vi "M2p_AD_Std_Simple.vi"() -> ()   [LabVIEW 2015]
uses:
  spcm_library/spcm_gui_common.llb/element_device.ctl
  spcm_library/spcm_gui_m2p.llb/element_m2p_ad_std.ctl
  spcm_library/spcm_gui_m2p.llb/element_m2p_ai_channel.ctl
  spcm_library/spcm_gui_common.llb/element_mode.ctl
  spcm_library/spcm_gui_m2p.llb/element_m2p_clock.ctl
  spcm_library/spcm_gui_m2p.llb/element_m2p_ai_trigger.ctl
  spcm_library/spcm_gui_m2p.llb/element_m2p_ai_multi_purpose_io.ctl
  spcm_library/spcm_gui_common.llb/element_device_infos.ctl
panel:
  out "Device Infos":T1={"Device Name"="M4i.4451-Exp", "Serial Number"=1122.0, "Mem (MB)"=4096.0}
  out "Display Data":dbl[][](graph)
  in  "M2p AD Settings":T2={"AI Channel 0"={"Enable"=TRUE, "Input Range "=2, "Termination"=0, "Input Type"=0, "Offset"=0}, "AI Channel 1"={"Enable"=TRUE, "Input Range "=2, "Termination"=0, "Input Type"=0, "Offset"=0}, "AI Channel 2"={"Enable"=TRUE, "Input Range "=2, "Termination"=0, "Input Type"=0, "Offset"=0}, "AI Channel 3"={"Enable"=TRUE, "Input Range "=2, "Termination"=0, "Input Type"=0, "Offset"=0}, "AI Channel 4"={"Enable"=TRUE, "Input Range "=2, "Termination"=0, "Input Type"=0, "Offset"=0}, "AI Channel 5"={"Enable"=TRUE, "Input Range "=2, "Termination"=0, "Input Type"=0, "Offset"=0}, "AI Channel 6"={"Enable"=TRUE, "Input Range "=2, "Termination"=0, "Input Type"=0, "Offset"=0}, "AI Channel 7"={"Enable"=TRUE, "Input Range "=2, "Termination"=0, "Input Type"=0, "Offset"=0}, "Mode Setup"={"Mode"=0, "Mem"=16384, "Seg"=1024, "Post"=8192, "Pre"=32, "ABA"=16}, "Clock Settings"={"Clock Mode"=0, "Sampling Rate (kHz)"=10000.0, "Clock Output"=FALSE, "Termination"=FALSE, "Ref. Clock (MHz)"=10.0, "Threshold (mV)"=1500}, "Trigger Settings"={"Trigger Source"=0, "External Trigger"=0, "Level 0 Ext"=1500, "Ext Trig Term"=FALSE, "Channel Trigger"=0, "Level 0 Ch"=0, "Level 1 Ch"=0, "Trigger Delay (Samples)"=0}, "Multi Purpose IO Lines"={"X0 Mode"=0, "X1 Mode"=0, "X2 Mode"=0, "X3 Mode"=0, "X0 ASync Send Pulse"=FALSE, "X1 ASync Send Pulse"=FALSE, "X2 ASync Send Pulse"=FALSE, "X3 ASync Send Pulse"=FALSE, "X1 Trigger Mode"=0, "X2 Trigger Mode"=0, "X3 Trigger Mode"=0, "X1 Pulsewidth"=0, "X2 Pulsewidth"=0, "X3 Pulsewidth"=0, "ASync Read Button"=FALSE, "ASync Read"=0, "AI"=TRUE}} {"Multi Purpose IO Lines"."X3 Mode" items=["Disable", "Asynchronous Out", "Asynchronous In", "Trigger Out", "Trigger In", "Clock Out", "Digital In", "Show Run State", "Show Arm State", "Show Sync Arm State"]; "Multi Purpose IO Lines"."X2 Mode" items=["Disable", "Asynchronous Out", "Asynchronous In", "Trigger Out", "Trigger In", "Clock Out", "Digital In", "Show Run State", "Show Arm State", "Show Sync Arm State"]; "Multi Purpose IO Lines"."X3 Trigger Mode" items=["Pos. Edge", "Neg. Edge", "Any Edge", "High Level", "Low Level", "PW Long Pos.", "PW Long Neg.", "PW Short Pos.", "PW Short Neg."]; "Multi Purpose IO Lines"."X2 Trigger Mode" items=["Pos. Edge", "Neg. Edge", "Any Edge", "High Level", "Low Level", "PW Long Pos.", "PW Long Neg.", "PW Short Pos.", "PW Short Neg."]; "Multi Purpose IO Lines"."X1 Trigger Mode" items=["Pos. Edge", "Neg. Edge", "Any Edge", "High Level", "Low Level", "PW Long Pos.", "PW Long Neg.", "PW Short Pos.", "PW Short Neg."]; "Multi Purpose IO Lines"."X1 Mode" items=["Disable", "Asynchronous Out", "Asynchronous In", "Trigger Out", "Trigger In", "Clock Out", "Digital In", "Show Run State", "Show Arm State", "Show Sync Arm State"]; "Multi Purpose IO Lines"."X0 Mode" items=["Disable", "Asynchronous Out", "Trigger Out", "Clock Out", "Show Run State", "Show Arm State", "Show Sync Arm State"]; "Trigger Settings"."Channel Trigger" items=["None", "Pos. Edge", "Neg. Edge", "Any Edge", "Pos. Rearm", "Neg. Rearm", "Enter Window", "Leave Window", "In Win", "Out Win"]; "Trigger Settings"."External Trigger" items=["None", "Pos. Edge", "Neg. Edge", "Any Edge", "High Level", "Low Level"]; "Trigger Settings"."Trigger Source" items=["Software Trigger", "External Trigger", "Channel 0 Trigger", "Channel 1 Trigger", "Channel 2 Trigger", "Channel 3 Trigger", "Channel 4 Trigger", "Channel 5 Trigger", "Channel 6 Trigger", "Channel 7 Trigger"]; "Trigger Settings"."Trigger Delay (Samples)" max=65535 step=1; "Clock Settings"."Threshold (mV)" min=-5000 max=5000; "Clock Settings"."Clock Mode" items=["Internal Clock Quartz", "External Clock", "External Reference Clock"]; "Clock Settings"."Ref. Clock (MHz)" min=0.0 max=125000.0; "Clock Settings"."Sampling Rate (kHz)" min=1.0 max=5000000.0; "Mode Setup"."Mode" items=["Singleshot", "Multiple Recording", "Gated Sampling", "ABA Mode"]; "Mode Setup"."ABA" min=2 max=65535 step=1; "Mode Setup"."Post" min=4 step=4; "Mode Setup"."Mem" min=8 step=4; "Mode Setup"."Pre" min=4 max=8176 step=4; "Mode Setup"."Seg" min=8 step=4; "AI Channel 7"."Input Type" items=["Single-ended", "Differential"]; "AI Channel 7"."Termination" items=["1 MOhm", "50 Ohm"]; "AI Channel 7"."Input Range" items=["±200 mV", "±500 mV", "±1000 mV", "±2000 mV", "±5000 mV", "±10000 mV"]; "AI Channel 6"."Input Type" items=["Single-ended", "Differential"]; "AI Channel 6"."Termination" items=["1 MOhm", "50 Ohm"]; "AI Channel 6"."Input Range" items=["±200 mV", "±500 mV", "±1000 mV", "±2000 mV", "±5000 mV", "±10000 mV"]; "AI Channel 5"."Input Type" items=["Single-ended", "Differential"]; "AI Channel 5"."Termination" items=["1 MOhm", "50 Ohm"]; "AI Channel 5"."Input Range" items=["±200 mV", "±500 mV", "±1000 mV", "±2000 mV", "±5000 mV", "±10000 mV"]; "AI Channel 4"."Input Type" items=["Single-ended", "Differential"]; "AI Channel 4"."Termination" items=["1 MOhm", "50 Ohm"]; "AI Channel 4"."Input Range" items=["±200 mV", "±500 mV", "±1000 mV", "±2000 mV", "±5000 mV", "±10000 mV"]; "AI Channel 3"."Input Type" items=["Single-ended", "Differential"]; "AI Channel 3"."Termination" items=["1 MOhm", "50 Ohm"]; "AI Channel 3"."Input Range" items=["±200 mV", "±500 mV", "±1000 mV", "±2000 mV", "±5000 mV", "±10000 mV"]; "AI Channel 2"."Input Type" items=["Single-ended", "Differential"]; "AI Channel 2"."Termination" items=["1 MOhm", "50 Ohm"]; "AI Channel 2"."Input Range" items=["±200 mV", "±500 mV", "±1000 mV", "±2000 mV", "±5000 mV", "±10000 mV"]; "AI Channel 1"."Input Type" items=["Single-ended", "Differential"]; "AI Channel 1"."Termination" items=["1 MOhm", "50 Ohm"]; "AI Channel 1"."Input Range" items=["±200 mV", "±500 mV", "±1000 mV", "±2000 mV", "±5000 mV", "±10000 mV"]; "AI Channel 0"."Input Type" items=["Single-ended", "Differential"]; "AI Channel 0"."Termination" items=["1 MOhm", "50 Ohm"]; "AI Channel 0"."Input Range" items=["±200 mV", "±500 mV", "±1000 mV", "±2000 mV", "±5000 mV", "±10000 mV"]}
  in  "Device":T8 {"Device" items=["Card", "digitizerNETBOX"]}
  # "Type"
  # "Offset"
  # "Range"
  # "Term"
  # "Mode / Clock / Multi IO"
  # "Trigger"
  # "Mode"
  # "ASync Write"
  # "Trig-Mode"
  # "Trig-Pulsewidth"
  # "ASync Read"
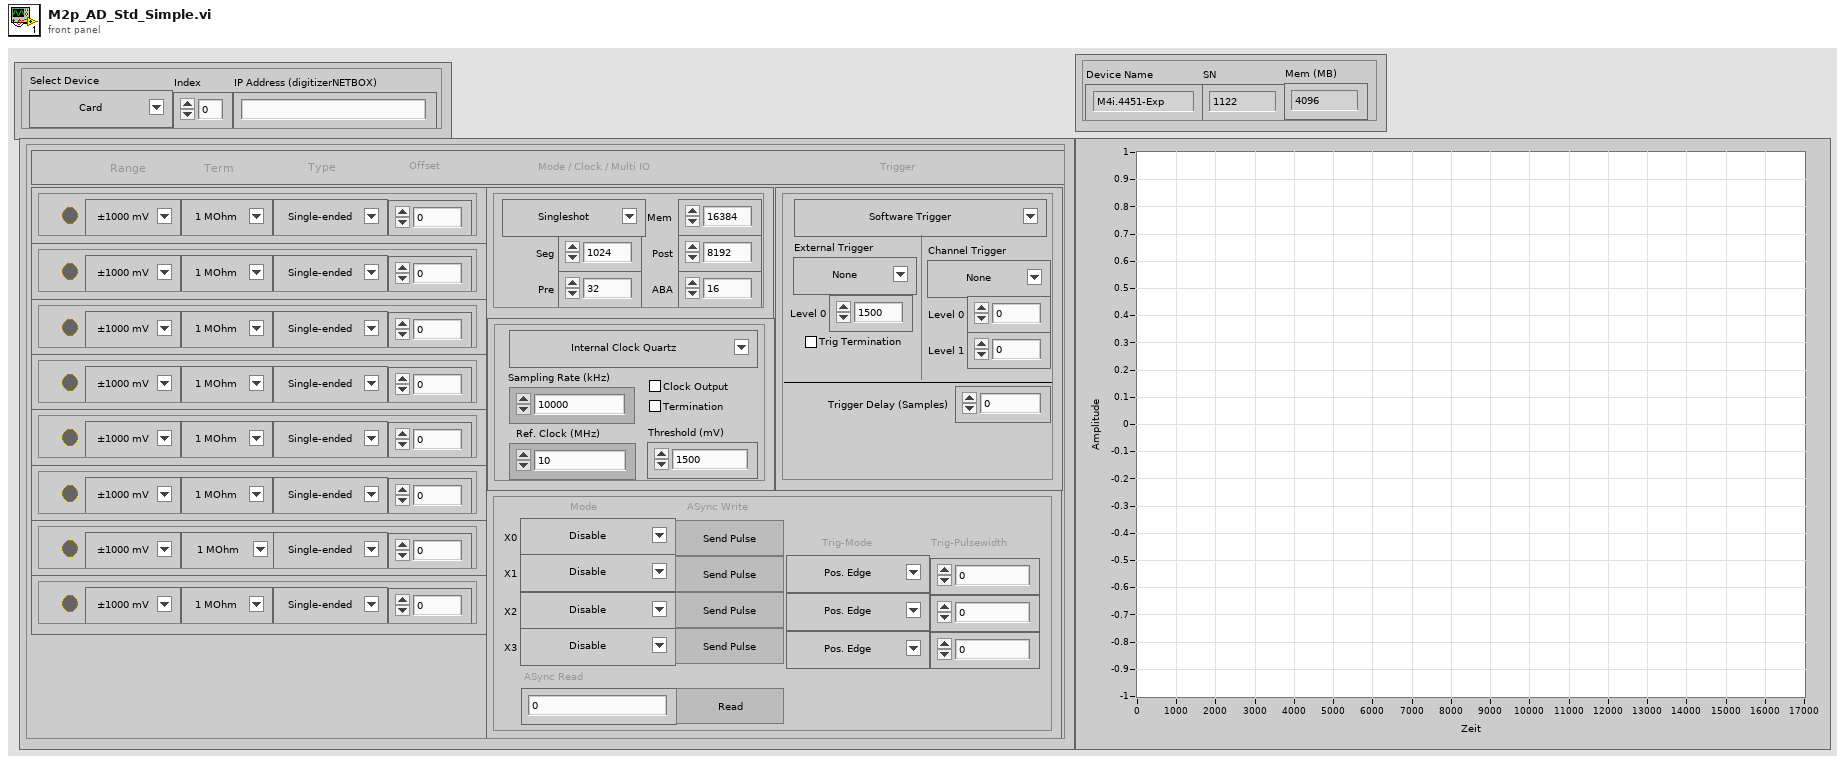
[diagram p1: front panel]
types:
  T1 = typedef "element_device_infos.ctl" = cluster{"Device Name":string, "Serial Number":dbl, "Mem (MB)":dbl}
  T2 = typedef "element_m2p_ad_std.ctl" = cluster{"AI Channel 0":T3, "AI Channel 1":T3, "AI Channel 2":T3, "AI Channel 3":T3, "AI Channel 4":T3, "AI Channel 5":T3, "AI Channel 6":T3, "AI Channel 7":T3, "Mode Setup":T4, "Clock Settings":T5, "Trigger Settings":T6, "Multi Purpose IO Lines":T7}
  T3 = typedef "element_m2p_ai_channel.ctl" = cluster{"Enable":bool, "Input Range ":u16, "Termination":u16, "Input Type":u16, "Offset":i32}
  T4 = typedef "element_mode.ctl" = cluster{"Mode":u16, "Mem":u32, "Seg":u32, "Post":u32, "Pre":u32, "ABA":u32}
  T5 = typedef "element_m2p_clock.ctl" = cluster{"Clock Mode":u16, "Sampling Rate (kHz)":dbl, "Clock Output":bool, "Termination":bool, "Ref. Clock (MHz)":dbl, "Threshold (mV)":i32}
  T6 = typedef "element_m2p_ai_trigger.ctl" = cluster{"Trigger Source":u16, "External Trigger":u16, "Level 0 Ext":i32, "Ext Trig Term":bool, "Channel Trigger":u16, "Level 0 Ch":i32, "Level 1 Ch":i32, "Trigger Delay (Samples)":u32}
  T7 = typedef "element_m2p_ai_multi_purpose_io.ctl" = cluster{"X0 Mode":u16, "X1 Mode":u16, "X2 Mode":u16, "X3 Mode":u16, "X0 ASync Send Pulse":bool, "X1 ASync Send Pulse":bool, "X2 ASync Send Pulse":bool, "X3 ASync Send Pulse":bool, "X1 Trigger Mode":u16, "X2 Trigger Mode":u16, "X3 Trigger Mode":u16, "X1 Pulsewidth":u32, "X2 Pulsewidth":u32, "X3 Pulsewidth":u32, "ASync Read Button":bool, "ASync Read":i32, "AI":bool}
  T8 = typedef "element_device.ctl" = cluster{"Index":dbl, "IP Address":string, "Device":u16}
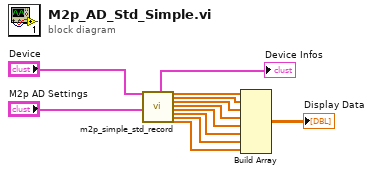
[diagram p0: block diagram]
diagram:
  n1 = call "m2p_simple_std_record.vi"("Device"="Device", "M2p AD Settings"="M2p AD Settings") -> ("Device Infos"=→"Device Infos":T1, "Ch0"=w9:dbl[], "Ch1"=w8:dbl[], "Ch2"=w7:dbl[], "Ch3"=w6:dbl[], "Ch4"=w5:dbl[], "Ch5"=w4:dbl[], "Ch6"=w3:dbl[], "Ch7"=w2:dbl[])  [unwired: 17 in]
  n2 = Build Array(w9, w8, w7, w6, w5, w4, w3, w2) -> (→"Display Data":dbl[][])
